vi "Get Rx Monitor Commands Section and Channels.vi"(8 "error in":errorcluster, 11 "custom device ref in":T1 format="%.0x") -> (0 "error out":errorcluster, 1 "Rx monitor section channel refs":T1[](array[typedef]) format="%.0x", 2 "Rx monitor section ref out":T1 format="%.0x", 3 "custom device ref out":T1 format="%.0x", 4 "found?":bool)   [LabVIEW 2020, in "AIM ARINC 664 Scripting.lvlib"]
uses:
  AIM ARINC 664 Scripting.lvlib
  Constants.vi
  <vilib>/NI VeriStand/Custom Device API/Custom Device Item Ref.ctl
  <vilib>/NI VeriStand/Custom Device API/Custom Device API.lvlib
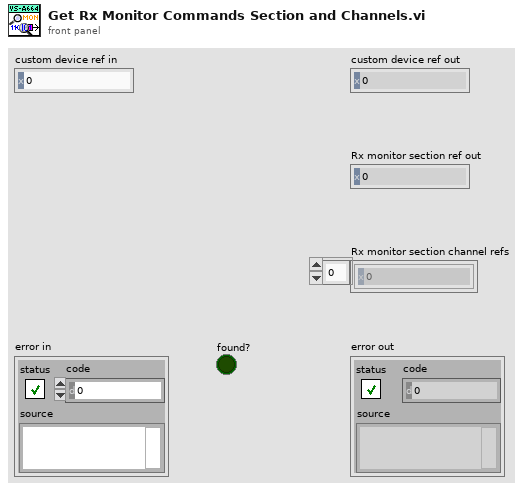
[diagram p1: front panel]
types:
  T1 = typedef "Custom Device API.lvlib/Custom Device Item Ref.ctl" = u64
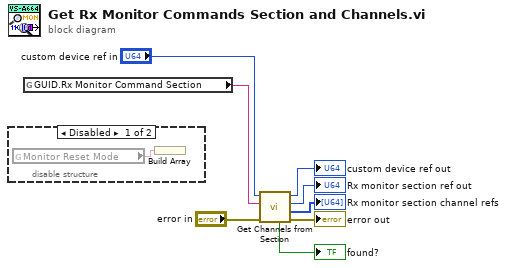
[diagram p0: block diagram]
diagram:
  n1 = disable-structure shown="Disabled" {
    frame Disabled {
      n2 = global read "Constants.vi" "Monitor Reset Mode"() -> (w9:string)
      n3 = Build Array(w9) -> ()  [unwired: 1 out]
    }
    frame Enabled {
    }
  }
  n4 = global read "Constants.vi" "GUID.Rx Monitor Command Section"() -> (w8:string)
  n5 = call "Get Channels from Section.vi"("error in"="error in", "GUID section"=w8, "custom device ref in"="custom device ref in") -> ("error out"=→"error out":errorcluster, "channel array refs out"=→"Rx monitor section channel refs":T1[], "section ref out"=→"Rx monitor section ref out":T1, "custom device ref out"=→"custom device ref out":T1, "all channels found?"=→"found?":bool)  [unwired: 3 in, 1 out]
